vi "OAT Extract Order Waveforms (Single Order).vi"(0 "scaled signal [EU]":waveform(dbl)={"t0"=timestamp(0 s since 1904-01-01), "dt"=0.0, "Y"=[]}, 5 "speed profile":T3 {"speed [RPM]" format="%.2f"; "time [s]" format="%.2f"}, 9 "orders to extract":dbl[](array[numeric])=[1.0] format="%.2f", 11 "error in (no error)":errorcluster, 12 "bandwidth":T2={"bandwidth value"=0.5, "bandwidth unit"=enum."Order"} {"bandwidth value" min=0.0 format="%.2f"}, 13 "window info":T1={"window type"=62, "window length"=2048} {"window type" items=["None"=0, "Hanning"=1, "Hamming"=2, "Blackman-Harris"=3, "Exact Blackman"=4, "Blackman"=5, "Flat Top"=6, "4 Term B-Harris"=7, "7 Term B-Harris"=8, "Low Sidelobe"=9, "Gaussian"=62]; "window length" min=0}) -> (4 "order waveforms [EU]":waveform(dbl)[](array[waveform]), 10 "unit label":string, 14 "actual window info":T1={"window type"=10, "window length"=2048} {"window type" items=["None"=0, "Hanning"=1, "Hamming"=2, "Blackman-Harris"=3, "Exact Blackman"=4, "Blackman"=5, "Flat Top"=6, "4 Term B-Harris"=7, "7 Term B-Harris"=8, "Low Sidelobe"=9, "Gaussian"=62]; "window length" min=0}, 15 "error out":errorcluster)   [LabVIEW 2017, in "SoundVib_Gabor.lvlib"]
doc: "Extracts order waveforms from specified orders in the <B>scaled signal [EU]</B>. This VI can return order waveforms of a single order or combined orders. Use <B>orders to extract</B> to specify the desired orders. This VI does not maintain state internally; you can use this VI in a loop to process multiple blocks. Wire data to the <B>scaled signal [EU]</B> input to determine the polymorphic instance to use or manually select the instance."
uses:
  <vilib>/addons/Sound and Vibration/Order Analysis/Gabor Order Tracking/SoundVib_Gabor.lvlib
  <vilib>/addons/Sound and Vibration/Order Analysis/Tach Process/SubVIs/speed profile.ctl
  <vilib>/addons/Sound and Vibration/Order Analysis/Ref Gabor Order Tracking/Mask Bandwidth.ctl
  <vilib>/addons/Sound and Vibration/Order Analysis/Ref Gabor Order Tracking/window information.ctl
  <vilib>/addons/_NISVFA/_Shared subVIs/Common/svc_Engineering Units to Unit Label.vi
  <vilib>/addons/_NISVFA/_Shared subVIs/Common/svc_Unit Label to Engineering Units.vi
  <vilib>/addons/Sound and Vibration/Order Analysis/Tach Process/SoundVib_TachProcess.lvlib
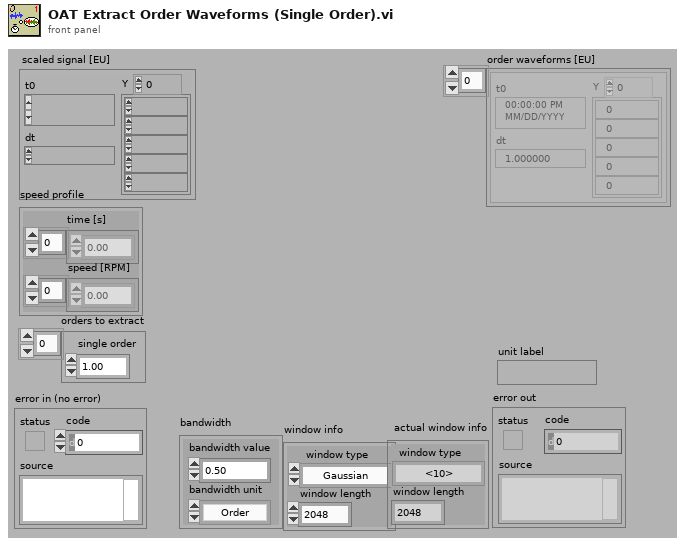
[diagram p1: front panel]
types:
  T1 = typedef "SoundVib_Gabor.lvlib/window information.ctl" = cluster{"window type":u32, "window length":i32}
  T2 = typedef "SoundVib_Gabor.lvlib/Mask Bandwidth.ctl" = cluster{"bandwidth value":dbl, "bandwidth unit":enum16{"Order", "Hz"}}
  T3 = typedef "SoundVib_TachProcess.lvlib/speed profile.ctl" = cluster{"time [s]":dbl[], "speed [RPM]":dbl[]}
  T4 = typedef "svc_Channel Info.ctl" = cluster{"sensor sensitivity":dbl, "engineering units":T5, "dB reference":dbl, "custom label":string, "weighting filter":T6, "pregain":dbl}
  T5 = typedef "svc_Engineering Units Text Ring.ctl" = u16
  T6 = typedef "svc_Weighting Filter Text Ring.ctl" = u16
  T7 = typedef "SoundVib_Gabor.lvlib/GT RefNum.ctl" = refnum<k1>
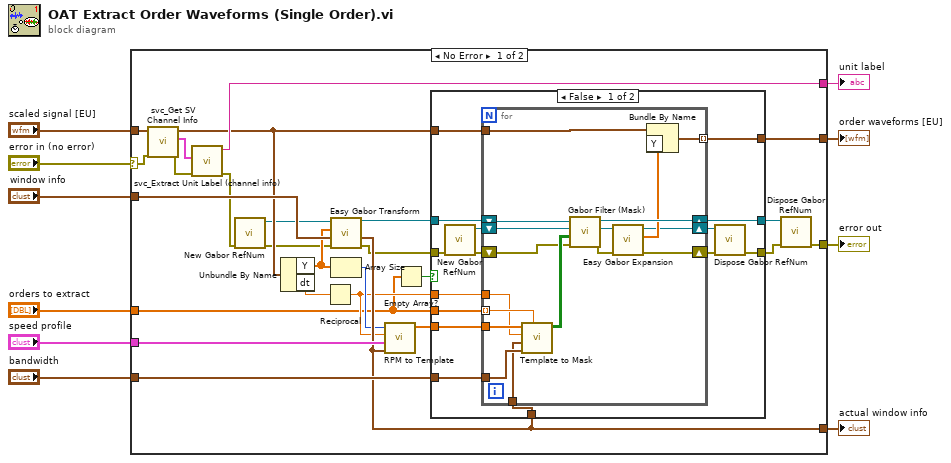
[diagram p0: block diagram]
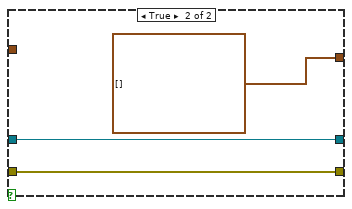
[diagram p2: hidden frame]
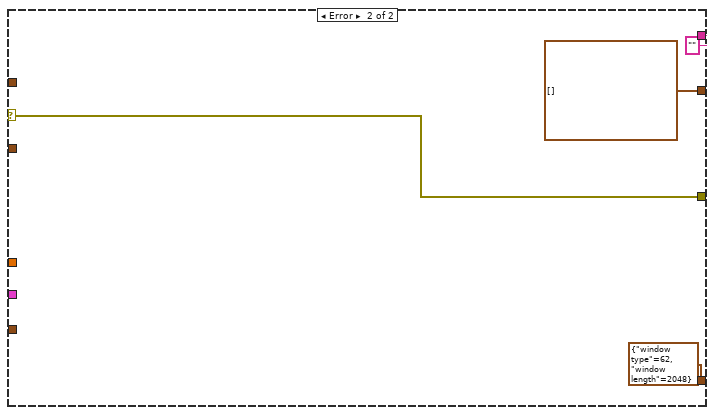
[diagram p3: hidden frame]
diagram:
  n1 = case shown="No Error" "error in (no error)" {
    selector: "error in (no error)" -> [w32 w75]
    tunnel: [w36 w75] -> w10
    tunnel: "speed profile" -> [w35 _]
    tunnel: [w34 waveform(dbl)[] []] -> w8
    tunnel: "scaled signal [EU]" -> [w33 _]
    tunnel: [w31 "" ("unit label")] -> w5
    tunnel: "window info" -> [w30 _]
    tunnel: "orders to extract" -> [w13 _]
    tunnel: "bandwidth" -> [w29 _]
    tunnel: [w28 T1 {"window type"=62, "window length"=2048} ("actual window")] -> w1
    frame No Error {
      n2 = call <vilib>:"svc_Get SV Channel Info.vi"("error in (no error)"=w32, "scaled signal [EU]"=w33) -> ("error out"=w16:errorcluster, "channel info"=w22:T4, "dup scaled signal [EU]"=w23:waveform(dbl))  [unwired: 4 in, 3 out]
      n3 = call <vilib>:"svc_Extract Unit Label (channel info).vi"("error in (no error)"=w16, "channel info"=w22) -> ("error out"=w15:errorcluster, "unit label"=w31:string)  [unwired: 7 in, 1 out]
      n4 = call <vilib>:"New Gabor RefNum.vi"("error in (no error)"=w15) -> ("error out"=w18:errorcluster, "RefNum"=w20:T7)  [unwired: 8 in]
      n5 = Unbundle By Name(w23) -> ("Y"=w19:dbl[], "dt"=w24:dbl)
      n6 = Reciprocal(x=w24) -> (1/x=w25:dbl)
      n7 = call <vilib>:"Easy Gabor Transform.vi"("error in (no error)"=w18, "window info"=w30, "x[n]"=w19, "RefNum in"=w20) -> ("error out"=w12:errorcluster, "actual window"=w28:T1, "RefNum out"=w17:T7)  [unwired: 3 in, 2 out]
      n8 = Array Size(array=w19) -> (size(s)=w26:i32)
      n9 = call <vilib>:"RPM to Template.vi"("window info"=w28, "speed profile"=w35, "sampling frequency [Hz]"=w25, "signal length"=w26) -> ("Gabor template"=w27:dbl[])  [unwired: 6 in, 1 out]
      n10 = Empty Array?(array=w13) -> (empty?=w14:bool)
      n11 = case shown="False" w14 {
        tunnel: [w51 waveform(dbl)[] []] -> w34
        tunnel: w13 -> [w50 _]
        tunnel: w29 -> [w49 _]
        tunnel: w28 -> [w48 _]
        tunnel: w27 -> [w47 _]
        tunnel: [w39 w69] -> w11
        tunnel: w25 -> [w46 _]
        tunnel: w23 -> [w45 _]
        tunnel: [w37 w71] -> w21
        tunnel: w17 -> [w44 w71]
        tunnel: w12 -> [w43 w69]
        frame False {
          n12 = call <vilib>:"New Gabor RefNum.vi"("error in (no error)"=w43) -> ("error out"=w41:errorcluster, "RefNum"=w42:T7)  [unwired: 8 in]
          n13 = for {
            tunnel: w47 -> [w65]
            tunnel: w50 -> [w63] mode=indexing
            shift-right: [w52] -> w40
            shift-left: w41 -> [w62]
            tunnel: [w53] -> w51 mode=indexing
            tunnel: w49 -> [w58]
            tunnel: w46 -> [w59]
            tunnel: w45 -> [w57]
            tunnel: w48 -> [w55]
            shift-right: [w66] -> w37
            shift-left: w44 -> [w68]
            shift-right: [w54] -> w38
            shift-left: w42 -> [w67]
            n14 = call <vilib>:"Template to Mask.vi"("order (1.0)"=w63, "bandwidth"=w58, "window info"=w55, "sampling frequency [S/s]"=w59, "Gabor template"=w65) -> ("mask array"=w64:bool[][])  [unwired: 6 in]
            n15 = call <vilib>:"Gabor Filter (Mask).vi"("error in (no error)"=w62, "mask array"=w64, "dest RefNum in"=w67, "src RefNum in"=w68) -> ("error out"=w60:errorcluster, "dest RefNum out"=w61:T7, "RefNum out"=w66:T7)  [unwired: 5 in]
            n16 = call <vilib>:"Easy Gabor Expansion.vi"("error in (no error)"=w60, "RefNum in"=w61) -> ("error out"=w52:errorcluster, "time waveform"=w56:dbl[], "RefNum out"=w54:T7)  [unwired: 7 in]
            n17 = Bundle By Name(cluster=w57, "Y"=w56) -> (w53:waveform(dbl))
          }
          n18 = call <vilib>:"Dispose Gabor RefNum.vi"("error in (no error)"=w40, "RefNum in"=w38) -> ("error out"=w39:errorcluster)  [unwired: 6 in]
        }
        frame True {
        }
      }
      n19 = call <vilib>:"Dispose Gabor RefNum.vi"("error in (no error)"=w11, "RefNum in"=w21) -> ("error out"=w36:errorcluster)  [unwired: 6 in]
    }
    frame Error {
    }
  }
  "order waveforms [EU]" <- w8
  "error out" <- w10
  "unit label" <- w5
  "actual window info" <- w1
